vi "AOTF_NonLinCreateTasks.vi"(1 "LineOnOff":bool[](array[boolean]), 3 "AmplitudenNiveaus":dbl[](array[numeric]), 7 "error in (no error)":errorcluster, 8 "FastAxisSteps":dbl) -> (5 "405out":refnum<k21>, 10 "task 8":refnum<k21>, 12 "task 4":refnum<k21>, 13 "LineOnOff[5]":bool, 14 "task 2":refnum<k21>, 15 "LineOnOff[4]":bool, 16 "task 3":refnum<k21>, 17 "LineOnOff[3]":bool, 18 "task 6":refnum<k21>, 19 "LineOnOff[2]":bool, 20 "task1":refnum<k21>, 21 "LineOnOff[7]":bool, 22 "task5":refnum<k21>, 23 "LineOnOff[6]":bool, 24 "task 7":refnum<k21>, 25 "LineOnOff[0]":bool, 26 "LineOnOff[1]":bool, 27 "error out":errorcluster)   [LabVIEW 2011]
uses:
  Variables/405Pico.vi
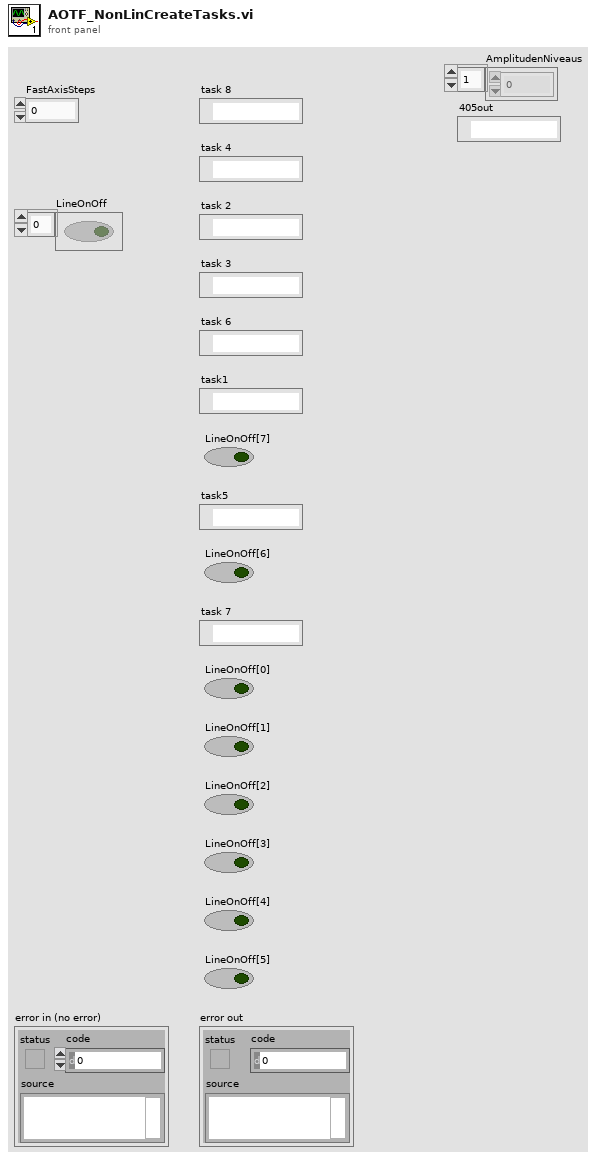
[diagram p1: front panel]
types:
  T1 = cluster{"LineOnOff[0]":bool, "LineOnOff[1]":bool, "LineOnOff[2]":bool, "LineOnOff[3]":bool, "LineOnOff[4]":bool, "LineOnOff[5]":bool, "LineOnOff[6]":bool, "LineOnOff[7]":bool, "LineOnOff[8]":bool}
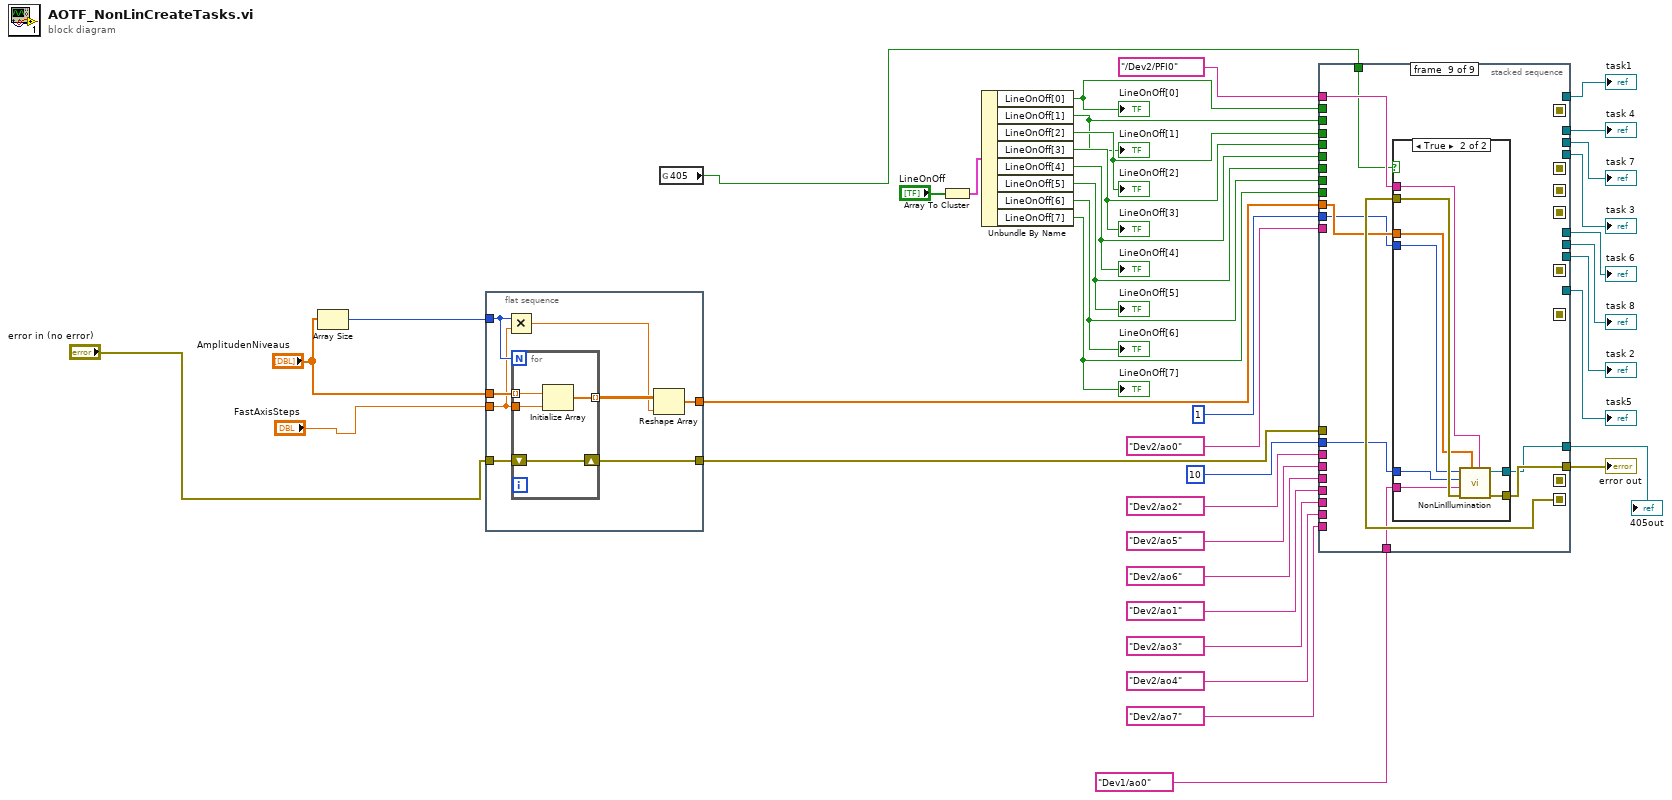
[diagram p0: block diagram]
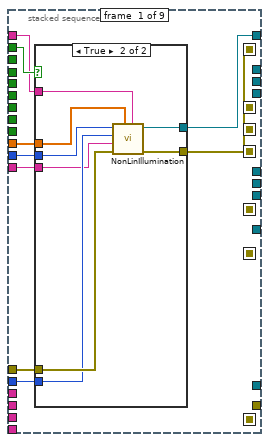
[diagram p2: hidden frame]
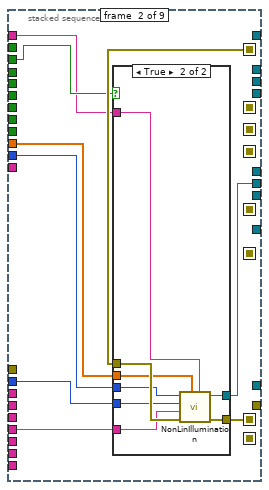
[diagram p4: hidden frame]
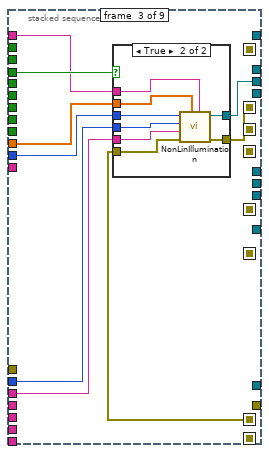
[diagram p6: hidden frame]
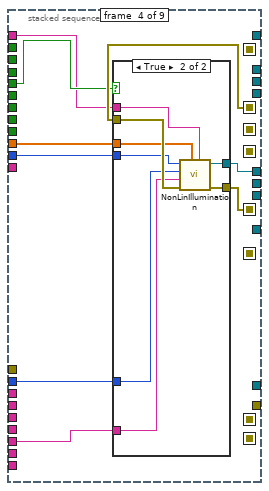
[diagram p8: hidden frame]
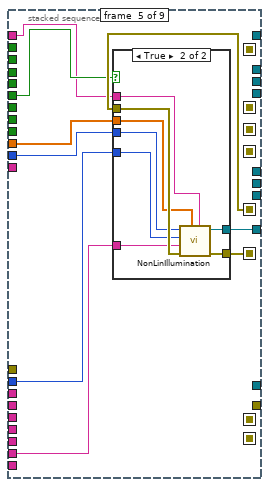
[diagram p10: hidden frame]
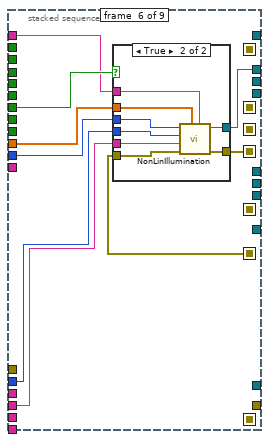
[diagram p12: hidden frame]
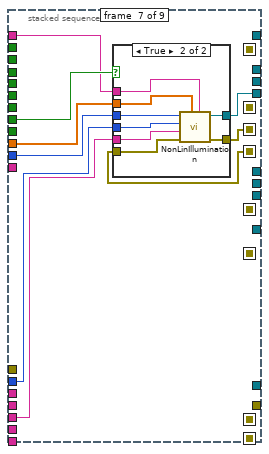
[diagram p14: hidden frame]
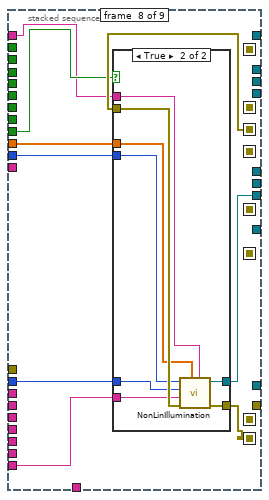
[diagram p16: hidden frame]
diagram:
  n1 = Array Size(array="AmplitudenNiveaus") -> (size(s)=w5:i32)
  n2 = flat-sequence {
    tunnel: "error in (no error)" -> [w47]
    tunnel: "FastAxisSteps" -> [w42]
    tunnel: [w45] -> w10
    tunnel: [w40] -> w9
    tunnel: "AmplitudenNiveaus" -> [w46]
    tunnel: w5 -> [w43]
    frame #0 {
      n3 = Multiply(x=w43, y=w42) -> (x*y=w41:dbl)
      n4 = for {
        N: w43 -> [_]
        tunnel: w46 -> [w51] mode=indexing
        shift-right: [w50] -> w45
        shift-left: w47 -> [w50]
        tunnel: w42 -> [w49]
        tunnel: [w48] -> w44 mode=indexing
        n5 = Initialize Array(w51, w49) -> (w48:dbl[])
      }
      n6 = Reshape Array(w44, w41) -> (w40:dbl[])
    }
  }
  n7 = global read "405Pico.vi" "405"() -> (w1:bool)
  n8 = Array To Cluster(array="LineOnOff") -> (cluster=w22:T1)
  n9 = Unbundle By Name(w22) -> ("LineOnOff[0]"=w23:bool, "LineOnOff[1]"=w24:bool, "LineOnOff[2]"=w25:bool, "LineOnOff[3]"=w26:bool, "LineOnOff[4]"=w27:bool, "LineOnOff[5]"=w28:bool, "LineOnOff[6]"=w29:bool, "LineOnOff[7]"=w30:bool)
  "LineOnOff[7]" <- w30
  "LineOnOff[6]" <- w29
  "LineOnOff[5]" <- w28
  "LineOnOff[4]" <- w27
  "LineOnOff[3]" <- w26
  "LineOnOff[2]" <- w25
  "LineOnOff[1]" <- w24
  "LineOnOff[0]" <- w23
  n10 = stacked-sequence {
    seq-local: [w59 _ _ _ _ _ _ _ _] -> [_ w78 _ _ _ _ _ _ _]
    seq-local: [_ w77 _ _ _ _ _ _ _] -> [_ _ w96 _ _ _ _ _ _]
    seq-local: [_ _ w95 _ _ _ _ _ _] -> [_ _ _ w114 _ _ _ _ _]
    seq-local: [_ _ _ w113 _ _ _ _ _] -> [_ _ _ _ w132 _ _ _ _]
    seq-local: [_ _ _ _ w131 _ _ _ _] -> [_ _ _ _ _ w150 _ _ _]
    seq-local: [_ _ _ _ _ w149 _ _ _] -> [_ _ _ _ _ _ w168 _ _]
    seq-local: [_ _ _ _ _ _ w167 _ _] -> [_ _ _ _ _ _ _ w186 _]
    seq-local: [_ _ _ _ _ _ _ w178 _] -> [_ _ _ _ _ _ _ _ w204]
    tunnel: w10 -> [w60 _ _ _ _ _ _ _ _]
    tunnel: [_ _ _ _ _ _ _ _ w198] -> w11
    tunnel: 1 -> [w58 w76 w94 w112 w130 w148 w166 w185 w202]
    tunnel: 10 -> [w57 w75 w93 w111 w129 w147 w165 w184 w200]
    tunnel: tag "Dev2/ao0" ("physical channels") -> [w56 _ _ _ _ _ _ _ _]
    tunnel: tag "Dev2/ao1" ("physical channels") -> [_ w74 _ _ _ _ _ _ _]
    tunnel: tag "Dev2/ao2" ("physical channels") -> [_ _ w92 _ _ _ _ _ _]
    tunnel: tag "Dev2/ao3" ("physical channels") -> [_ _ _ w110 _ _ _ _ _]
    tunnel: tag "Dev2/ao4" ("physical channels") -> [_ _ _ _ w128 _ _ _ _]
    tunnel: tag "Dev2/ao5" ("physical channels") -> [_ _ _ _ _ w146 _ _ _]
    tunnel: tag "Dev2/ao6" ("physical channels") -> [_ _ _ _ _ _ w164 _ _]
    tunnel: tag "Dev2/ao7" ("physical channels") -> [_ _ _ _ _ _ _ w183 _]
    tunnel: w23 -> [w55 _ _ _ _ _ _ _ _]
    tunnel: w24 -> [_ w73 _ _ _ _ _ _ _]
    tunnel: w25 -> [_ _ w91 _ _ _ _ _ _]
    tunnel: w26 -> [_ _ _ w109 _ _ _ _ _]
    tunnel: w27 -> [_ _ _ _ w127 _ _ _ _]
    tunnel: w28 -> [_ _ _ _ _ w145 _ _ _]
    tunnel: w29 -> [_ _ _ _ _ _ w163 _ _]
    tunnel: w30 -> [_ _ _ _ _ _ _ w182 _]
    tunnel: [w54 _ _ _ _ _ _ _ _] -> w32
    tunnel: [_ w72 _ _ _ _ _ _ _] -> w33
    tunnel: [_ _ w90 _ _ _ _ _ _] -> w34
    tunnel: [_ _ _ w108 _ _ _ _ _] -> w35
    tunnel: [_ _ _ _ w126 _ _ _ _] -> w36
    tunnel: [_ _ _ _ _ w144 _ _ _] -> w37
    tunnel: [_ _ _ _ _ _ w162 _ _] -> w38
    tunnel: [_ _ _ _ _ _ _ w181 _] -> w39
    tunnel: w9 -> [w53 w71 w89 w107 w125 w143 w161 w180 w203]
    tunnel: tag "/Dev2/PFI0" ("TriggerStart") -> [w52 w70 w88 w106 w124 w142 w160 w179 w201]
    tunnel: tag "Dev1/ao0" ("physical channels") -> [_ _ _ _ _ _ _ _ w199]
    tunnel: [_ _ _ _ _ _ _ _ w197] -> w2
    tunnel: w1 -> [_ _ _ _ _ _ _ _ w196]
    frame #0 {
      n11 = case shown="True" w55 {
        tunnel: w60 -> [w61 w69]
        tunnel: [w61 w68] -> w59
        tunnel: w58 -> [_ w67]
        tunnel: w57 -> [_ w66]
        tunnel: w56 -> [_ w65]
        tunnel: [_ w64] -> w54
        tunnel: w53 -> [_ w63]
        tunnel: w52 -> [_ w62]
        frame False {
        }
        frame True {
          n12 = call "NonLinIllumination.vi"("TriggerStart"=w62, "array curve"=w63, "error in (no error)"=w69, "physical channels"=w65, "maximum value"=w66, "minimum value"=w67) -> ("error out"=w68:errorcluster, "task out"=w64:refnum<k21>)  [unwired: 4 in]
        }
      }
    }
    frame #1 {
      n13 = case shown="True" w73 {
        tunnel: w78 -> [w79 w87]
        tunnel: [w79 w86] -> w77
        tunnel: w76 -> [_ w85]
        tunnel: w75 -> [_ w84]
        tunnel: w74 -> [_ w83]
        tunnel: [_ w82] -> w72
        tunnel: w71 -> [_ w81]
        tunnel: w70 -> [_ w80]
        frame False {
        }
        frame True {
          n14 = call "NonLinIllumination.vi"("TriggerStart"=w80, "array curve"=w81, "error in (no error)"=w87, "physical channels"=w83, "maximum value"=w84, "minimum value"=w85) -> ("error out"=w86:errorcluster, "task out"=w82:refnum<k21>)  [unwired: 4 in]
        }
      }
    }
    frame #2 {
      n15 = case shown="True" w91 {
        tunnel: w96 -> [w97 w105]
        tunnel: [w97 w104] -> w95
        tunnel: w94 -> [_ w103]
        tunnel: w93 -> [_ w102]
        tunnel: w92 -> [_ w101]
        tunnel: [_ w100] -> w90
        tunnel: w89 -> [_ w99]
        tunnel: w88 -> [_ w98]
        frame False {
        }
        frame True {
          n16 = call "NonLinIllumination.vi"("TriggerStart"=w98, "array curve"=w99, "error in (no error)"=w105, "physical channels"=w101, "maximum value"=w102, "minimum value"=w103) -> ("error out"=w104:errorcluster, "task out"=w100:refnum<k21>)  [unwired: 4 in]
        }
      }
    }
    frame #3 {
      n17 = case shown="True" w109 {
        tunnel: w114 -> [w115 w123]
        tunnel: [w115 w122] -> w113
        tunnel: w112 -> [_ w121]
        tunnel: w111 -> [_ w120]
        tunnel: w110 -> [_ w119]
        tunnel: [_ w118] -> w108
        tunnel: w107 -> [_ w117]
        tunnel: w106 -> [_ w116]
        frame False {
        }
        frame True {
          n18 = call "NonLinIllumination.vi"("TriggerStart"=w116, "array curve"=w117, "error in (no error)"=w123, "physical channels"=w119, "maximum value"=w120, "minimum value"=w121) -> ("error out"=w122:errorcluster, "task out"=w118:refnum<k21>)  [unwired: 4 in]
        }
      }
    }
    frame #4 {
      n19 = case shown="True" w127 {
        tunnel: w132 -> [w133 w141]
        tunnel: [w133 w140] -> w131
        tunnel: w130 -> [_ w139]
        tunnel: w129 -> [_ w138]
        tunnel: w128 -> [_ w137]
        tunnel: [_ w136] -> w126
        tunnel: w125 -> [_ w135]
        tunnel: w124 -> [_ w134]
        frame False {
        }
        frame True {
          n20 = call "NonLinIllumination.vi"("TriggerStart"=w134, "array curve"=w135, "error in (no error)"=w141, "physical channels"=w137, "maximum value"=w138, "minimum value"=w139) -> ("error out"=w140:errorcluster, "task out"=w136:refnum<k21>)  [unwired: 4 in]
        }
      }
    }
    frame #5 {
      n21 = case shown="True" w145 {
        tunnel: w150 -> [w151 w159]
        tunnel: [w151 w158] -> w149
        tunnel: w148 -> [_ w157]
        tunnel: w147 -> [_ w156]
        tunnel: w146 -> [_ w155]
        tunnel: [_ w154] -> w144
        tunnel: w143 -> [_ w153]
        tunnel: w142 -> [_ w152]
        frame False {
        }
        frame True {
          n22 = call "NonLinIllumination.vi"("TriggerStart"=w152, "array curve"=w153, "error in (no error)"=w159, "physical channels"=w155, "maximum value"=w156, "minimum value"=w157) -> ("error out"=w158:errorcluster, "task out"=w154:refnum<k21>)  [unwired: 4 in]
        }
      }
    }
    frame #6 {
      n23 = case shown="True" w163 {
        tunnel: w168 -> [w169 w177]
        tunnel: [w169 w176] -> w167
        tunnel: w166 -> [_ w175]
        tunnel: w165 -> [_ w174]
        tunnel: w164 -> [_ w173]
        tunnel: [_ w172] -> w162
        tunnel: w161 -> [_ w171]
        tunnel: w160 -> [_ w170]
        frame False {
        }
        frame True {
          n24 = call "NonLinIllumination.vi"("TriggerStart"=w170, "array curve"=w171, "error in (no error)"=w177, "physical channels"=w173, "maximum value"=w174, "minimum value"=w175) -> ("error out"=w176:errorcluster, "task out"=w172:refnum<k21>)  [unwired: 4 in]
        }
      }
    }
    frame #7 {
      n25 = case shown="True" w182 {
        tunnel: w186 -> [w187 w195]
        tunnel: [w187 w194] -> w178
        tunnel: w185 -> [_ w193]
        tunnel: w184 -> [_ w192]
        tunnel: w183 -> [_ w191]
        tunnel: [_ w190] -> w181
        tunnel: w180 -> [_ w189]
        tunnel: w179 -> [_ w188]
        frame False {
        }
        frame True {
          n26 = call "NonLinIllumination.vi"("TriggerStart"=w188, "array curve"=w189, "error in (no error)"=w195, "physical channels"=w191, "maximum value"=w192, "minimum value"=w193) -> ("error out"=w194:errorcluster, "task out"=w190:refnum<k21>)  [unwired: 4 in]
        }
      }
    }
    frame #8 {
      n27 = case shown="True" w196 {
        tunnel: w204 -> [w205 w213]
        tunnel: [w205 w212] -> w198
        tunnel: w202 -> [_ w211]
        tunnel: w200 -> [_ w210]
        tunnel: w199 -> [_ w209]
        tunnel: [_ w208] -> w197
        tunnel: w203 -> [_ w207]
        tunnel: w201 -> [_ w206]
        frame False {
        }
        frame True {
          n28 = call "NonLinIllumination.vi"("TriggerStart"=w206, "array curve"=w207, "error in (no error)"=w213, "physical channels"=w209, "maximum value"=w210, "minimum value"=w211) -> ("error out"=w212:errorcluster, "task out"=w208:refnum<k21>)  [unwired: 4 in]
        }
      }
    }
  }
  "task 2" <- w39
  "task 3" <- w38
  "task 4" <- w37
  "task5" <- w36
  "task 6" <- w35
  "task 7" <- w34
  "task 8" <- w33
  "task1" <- w32
  "error out" <- w11
  "405out" <- w2
